vi "refValueToTriggerEvent.vi"() -> ()   [LabVIEW 2015]
panel:
  out "data":T1(ring)
  in  "Change":bool=TRUE
  out "Numeric 2":i32
  out "Numeric":dbl
  in  "OK Button 16":bool
  in  "OK Button 15":bool
  in  "OK Button 14":bool
  in  "OK Button 13":bool
  in  "OK Button 12":bool
  in  "OK Button 11":bool
  in  "OK Button 10":bool
  in  "OK Button 9":bool
  in  "OK Button 8":bool
  in  "OK Button 7":bool
  in  "OK Button 6":bool
  in  "OK Button 5":bool
  in  "OK Button 4":bool
  in  "OK Button 3":bool
  in  "OK Button 2":bool
  in  "OK Button":bool
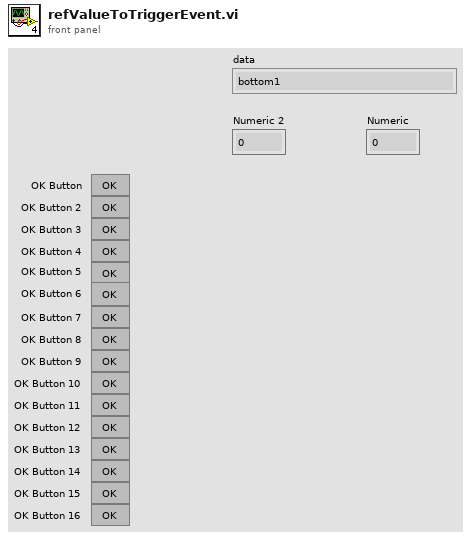
[diagram p1: front panel]
types:
  T1 = enum16{"bottom1", "bottom2", "bottom3", "bottom4", "bottom5", "bottom6", "bottom7", "bottom8", "bottom9", "bottom10", "bottom11", "bottom12", "bottom13", "bottom14", "bottom15", "bottom16"}
  T2 = cluster{"Value":bool, "Value":bool, "Value":bool, "Value":bool, "Value":bool, "Value":bool, "Value":bool, "Value":bool, "Value":bool, "Value":bool, "Value":bool, "Value":bool, "Value":bool, "Value":bool, "Value":bool, "Value":bool}
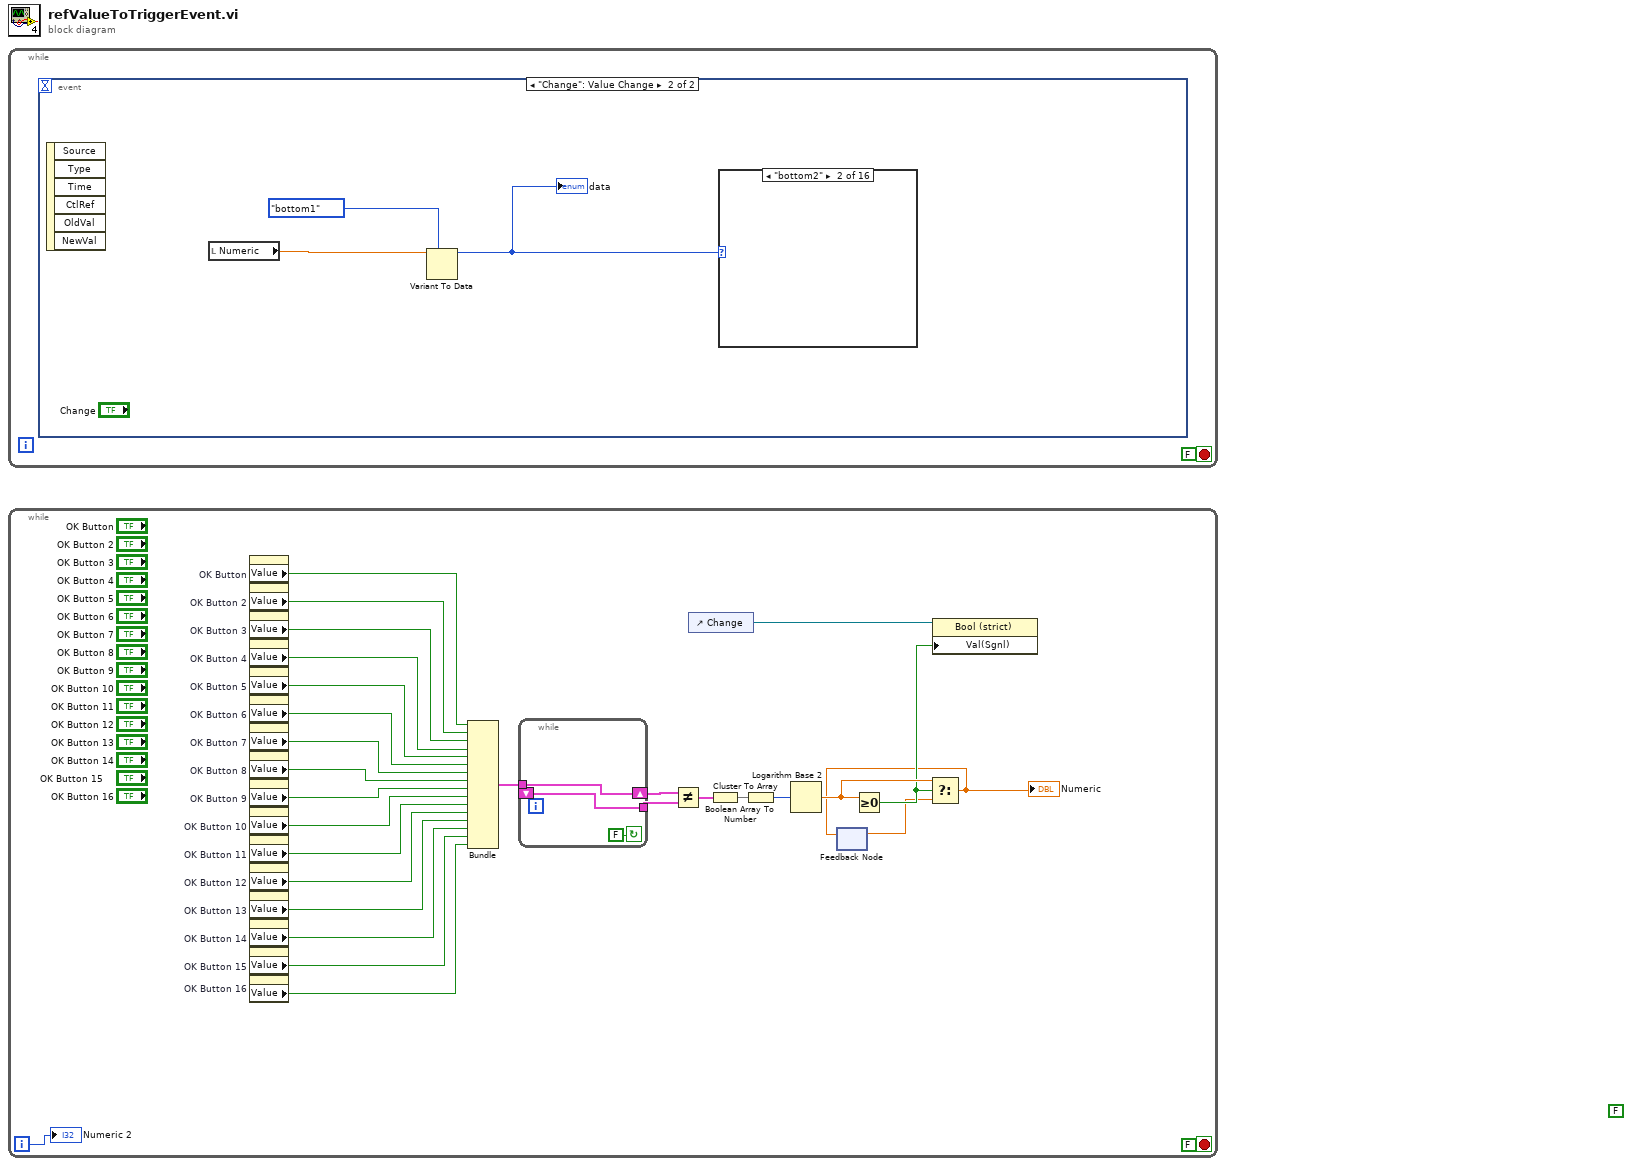
[diagram p0: block diagram]
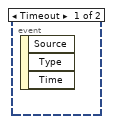
[diagram p2: hidden frame]
diagram:
  (unwired) FALSE
  n1 = while {
    stop <- FALSE stop-if-true
    n2 = event shown="[1] \"Change\": Value Change" {
      selector: _ -> [_ _]
      dyn-events: _ -> [_ _]
      timeout: _ -> [_ _]
      event Timeout {
        n3 = event-data() -> ()  [unwired: 1 in, 3 out]
      }
      event "Change": Value Change {
        n4 = event-data() -> ()  [unwired: 1 in, 6 out]
        n5 = local read "Numeric"() -> (w3:dbl)
        n6 = Variant To Data(type=T1."bottom1" ("Enum"), Variant=w3) -> (data=w2:T1)  [unwired: 1 in, 1 out]
        "data" <- w2
        n7 = case shown="\"bottom2\"" w2 {
          frame "bottom1", Default {
          }
          frame "bottom2" {
          }
          frame "bottom3" {
          }
          frame "bottom4" {
          }
          frame "bottom5" {
          }
          frame "bottom6" {
          }
          frame "bottom7" {
          }
          frame "bottom8" {
          }
          frame "bottom9" {
          }
          frame "bottom10" {
          }
          frame "bottom11" {
          }
          frame "bottom12" {
          }
          frame "bottom13" {
          }
          frame "bottom14" {
          }
          frame "bottom15" {
          }
          frame "bottom16" {
          }
        }
      }
    }
  }
  n8 = while {
    i -> [w32]
    stop <- FALSE stop-if-true
    n9 = property on="OK Button" class="Bool (strict)"() -> ("Value"=w20:bool)  [unwired: 2 in, 2 out]
    n10 = property on="OK Button 2" class="Bool (strict)"() -> ("Value"=w19:bool)  [unwired: 2 in, 2 out]
    n11 = property on="OK Button 3" class="Bool (strict)"() -> ("Value"=w18:bool)  [unwired: 2 in, 2 out]
    n12 = property on="OK Button 4" class="Bool (strict)"() -> ("Value"=w17:bool)  [unwired: 2 in, 2 out]
    n13 = property on="OK Button 5" class="Bool (strict)"() -> ("Value"=w21:bool)  [unwired: 2 in, 2 out]
    n14 = property on="OK Button 6" class="Bool (strict)"() -> ("Value"=w22:bool)  [unwired: 2 in, 2 out]
    n15 = property on="OK Button 7" class="Bool (strict)"() -> ("Value"=w23:bool)  [unwired: 2 in, 2 out]
    n16 = property on="OK Button 8" class="Bool (strict)"() -> ("Value"=w16:bool)  [unwired: 2 in, 2 out]
    n17 = property on="OK Button 9" class="Bool (strict)"() -> ("Value"=w24:bool)  [unwired: 2 in, 2 out]
    n18 = property on="OK Button 10" class="Bool (strict)"() -> ("Value"=w25:bool)  [unwired: 2 in, 2 out]
    n19 = property on="OK Button 11" class="Bool (strict)"() -> ("Value"=w26:bool)  [unwired: 2 in, 2 out]
    n20 = property on="OK Button 12" class="Bool (strict)"() -> ("Value"=w27:bool)  [unwired: 2 in, 2 out]
    n21 = property on="OK Button 13" class="Bool (strict)"() -> ("Value"=w28:bool)  [unwired: 2 in, 2 out]
    n22 = property on="OK Button 14" class="Bool (strict)"() -> ("Value"=w29:bool)  [unwired: 2 in, 2 out]
    n23 = property on="OK Button 15" class="Bool (strict)"() -> ("Value"=w30:bool)  [unwired: 2 in, 2 out]
    n24 = property on="OK Button 16" class="Bool (strict)"() -> ("Value"=w31:bool)  [unwired: 2 in, 2 out]
    n25 = Bundle("Value"=w20, "Value"=w19, "Value"=w18, "Value"=w17, "Value"=w21, "Value"=w22, "Value"=w23, "Value"=w16, "Value"=w24, "Value"=w25, "Value"=w26, "Value"=w27, "Value"=w28, "Value"=w29, "Value"=w30, "Value"=w31) -> (w7:T2)  [unwired: 1 in]
    n26 = while {
      tunnel: w7 -> [w36]
      shift-right: [w36] -> w11
      shift-left: _ -> [w35]
      tunnel: [w35] -> w12
      stop <- FALSE continue-if-true
    }
    n27 = Not Equal?(x=w11, y=w12) -> (x != y?=w9:T2)
    n28 = control-ref of="Change"() -> (w6:refnum<vi>)
    n29 = Cluster To Array(cluster=w9) -> (array=w10:bool[])
    n30 = Boolean Array To Number(Boolean array=w10) -> (number=w8:u32)
    n31 = Logarithm Base 2(1:w8) -> (0:w15:dbl)
    n32 = feedback #1() -> (w13:dbl)  [unwired: 1 in]
    n33 = Greater Or Equal To 0?(x=w15) -> (x >= 0?=w14:bool)
    n34 = Select(t=w15, s=w14, f=w13) -> (s? t:f=w5:dbl)
    "Numeric" <- w5
    n35 = feedback-in #1(w5) -> ()
    n36 = property on="Property Node" class="Bool (strict)"(reference=w6, "Val(Sgnl)"=w14) -> ()  [unwired: 1 in, 2 out]
    "Numeric 2" <- w32
  }
